vi "Data_Write_Accum.vi"(7 "wfm info":T2, 8 "error in (no error)":errorcluster, 10 "QMH ICR Cluster":T1, 11 "data":i16[](array[numeric])) -> (0 "error out":errorcluster, 1 "Is Accumulated ?":bool, 2 "QMH ICR Cluster":T1, 3 "data":i16[](array[numeric]))   [LabVIEW 2024]
doc: "This VI writes an ACCUMULATED raw dataset to a disk file.\nIf number of accumulations is 1 (i.e. no accumulation), nothing is done, no disk file is created.\nIf number of accumulations > 1 (i.e Nacc > 1) :\n- during the first accumulation, the signal is divided by Nacc and stored into the accumulated disk file.\n- during the next accumulations, the signal is divided by Nacc, added to the previous accumulated signal, and stored into the disk file.\n- the final accumulated signal will contain (signal1 / Nacc + signal2 / Nacc + ... + signalNacc / Nacc)"
uses:
  controls/QMH_ICR_Cluster.ctl
  controls/HARDWARE_Resources.ctl
  controls/PROCESSING_Inputs.ctl
  controls/LOOPS_Inputs.ctl
  controls/OPO_Inputs.ctl
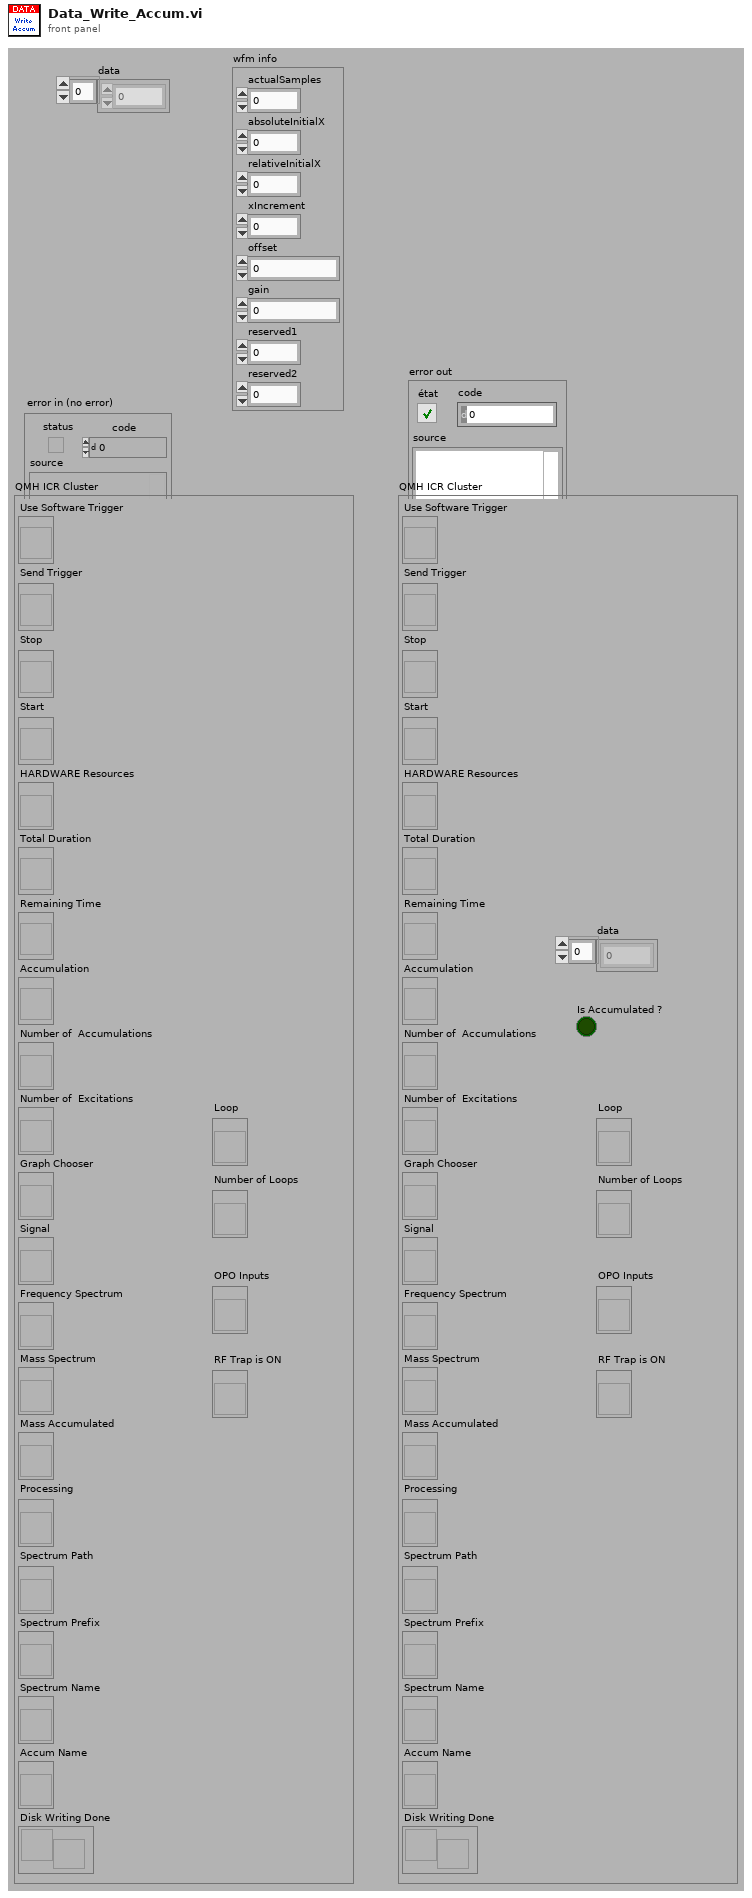
[diagram p1: front panel]
types:
  T1 = typedef "QMH_ICR_Cluster.ctl" = cluster{"Use Software Trigger":refnum<vi>, "Send Trigger":refnum<vi>, "Stop":refnum<vi>, "Start":refnum<vi>, "HARDWARE Resources":refnum<vi>, "Total Duration":refnum<vi>, "Remaining Time":refnum<vi>, "Accumulation":refnum<vi>, "Number of  Accumulations":refnum<vi>, "Number of  Excitations":refnum<vi>, "Graph Chooser":refnum<vi>, "Signal":refnum<vi>, "Frequency Spectrum":refnum<vi>, "Mass Spectrum":refnum<vi>, "Mass Accumulated":refnum<vi>, "Processing":refnum<vi>, "Spectrum Path":refnum<vi>, "Spectrum Prefix":refnum<vi>, "Spectrum Name":refnum<vi>, "Accum Name":refnum<vi>, "Disk Writing Done":refnum<notifier>, "Loop":refnum<vi>, "Number of Loops":refnum<vi>, "OPO Inputs":refnum<vi>, "RF Trap is ON":refnum<vi>}
  T2 = cluster{"actualSamples":i32, "absoluteInitialX":dbl, "relativeInitialX":dbl, "xIncrement":dbl, "offset":dbl, "gain":dbl, "reserved1":dbl, "reserved2":dbl}
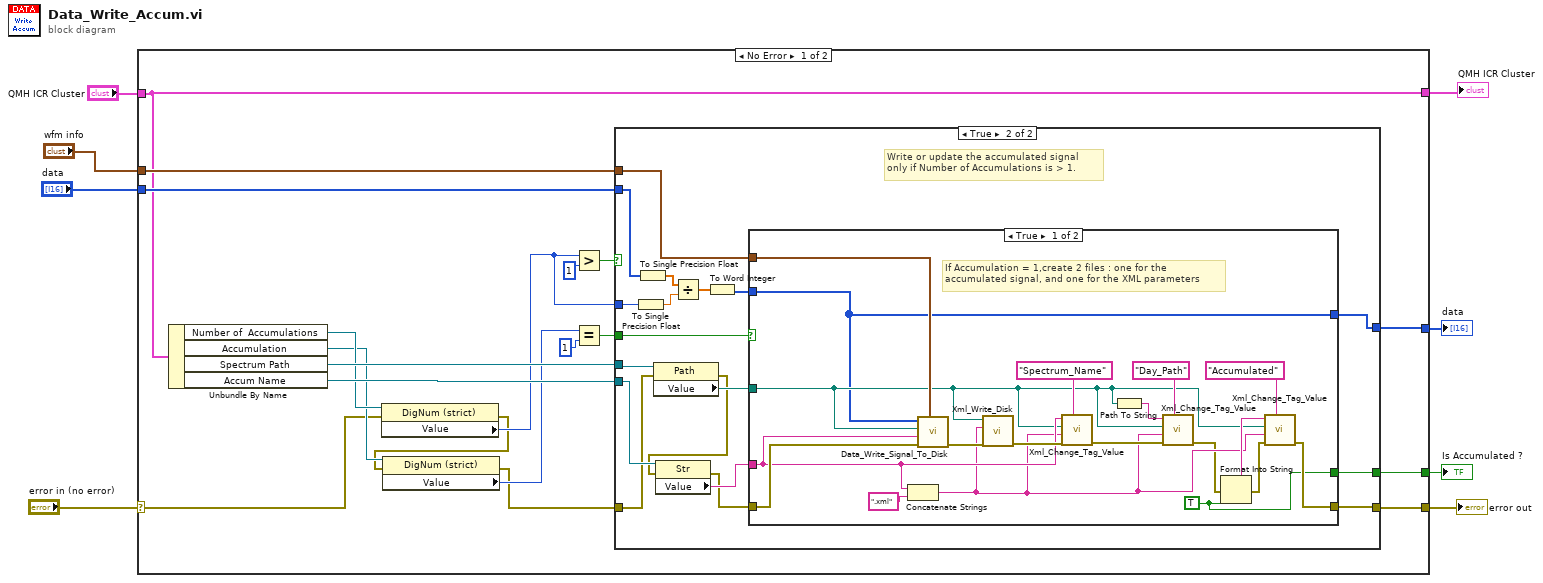
[diagram p0: block diagram]
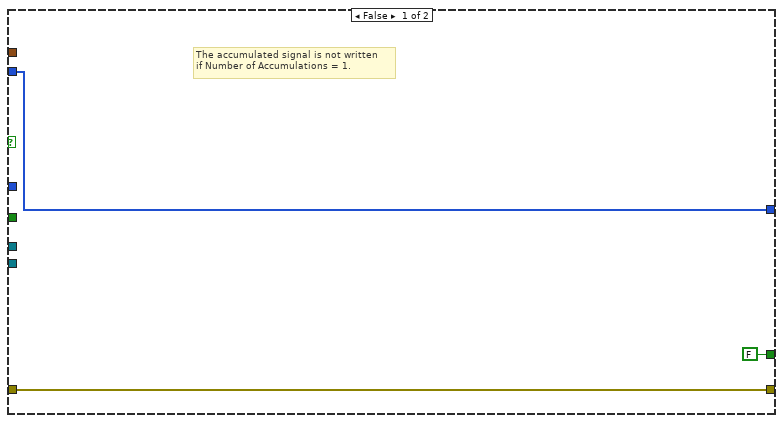
[diagram p2: hidden frame]
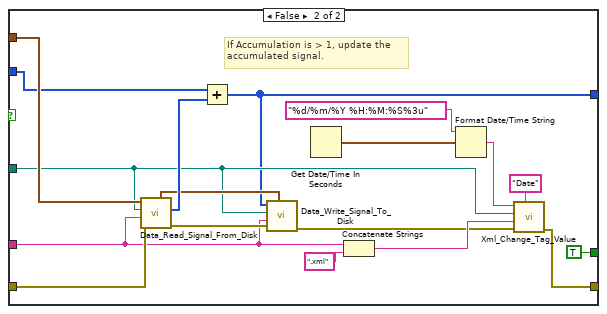
[diagram p3: hidden frame]
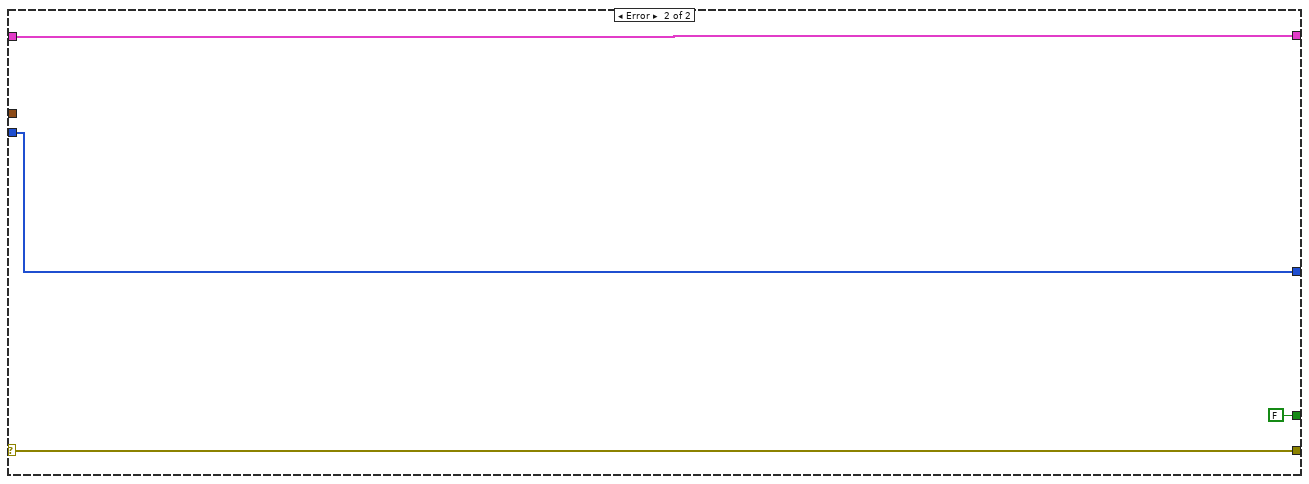
[diagram p4: hidden frame]
diagram:
  n1 = case shown="No Error" "error in (no error)" {
    selector: "error in (no error)" -> [w12 w89]
    tunnel: [w21 w89] -> w6
    tunnel: "wfm info" -> [w27 _]
    tunnel: "data" -> [w26 w87]
    tunnel: "QMH ICR Cluster" -> [w20 w88]
    tunnel: [w20 w88] -> w3
    tunnel: [w13 w87] -> w2
    tunnel: [w9 FALSE] -> w1
    frame No Error {
      n2 = Unbundle By Name(w20) -> ("Number of  Accumulations"=w19:refnum<vi>, "Accumulation"=w18:refnum<vi>, "Spectrum Path"=w25:refnum<vi>, "Accum Name"=w24:refnum<vi>)
      n3 = property class="DigNum (strict)"(reference=w19, error in=w12) -> (error out=w11:errorcluster, "Value"=w14:i16)  [unwired: 1 out]
      n4 = property class="DigNum (strict)"(reference=w18, error in=w11) -> (error out=w10:errorcluster, "Value"=w15:i16)  [unwired: 1 out]
      n5 = Greater?(x=w14, y=i16 1) -> (0:w23:bool)
      n6 = Equal?(x=w15, y=i16 1) -> (x = y?=w16:bool)
      n7 = case shown="True" w23 {
        tunnel: w27 -> [_ w42]
        tunnel: w26 -> [w29 w37]
        tunnel: w25 -> [_ w48]
        tunnel: w24 -> [_ w47]
        tunnel: w10 -> [w30 w40]
        tunnel: [w30 w44] -> w21
        tunnel: w16 -> [_ w43]
        tunnel: w14 -> [_ w41]
        tunnel: [w29 w31] -> w13
        tunnel: [FALSE w32] -> w9
        frame False {
          # "The accumulated signal is not written\nif Number of Accumulations = 1."
        }
        frame True {
          # "Write or update the accumulated signal\nonly if Number of Accumulations is > 1."
          n8 = To Single Precision Float(number=w41) -> (single precision float=w34:sgl)
          n9 = To Single Precision Float(number=w37) -> (single precision float=w35:sgl[])
          n10 = property class="Path"(reference=w48, error in=w40) -> (error out=w39:errorcluster, "Value"=w46:path)  [unwired: 1 out]
          n11 = property class="Str"(reference=w47, error in=w39) -> (error out=w38:errorcluster, "Value"=w45:string)  [unwired: 1 out]
          n12 = Divide(x=w35, y=w34) -> (x/y=w36:sgl[])
          n13 = To Word Integer(number=w36) -> (16bit integer=w33:i16[])
          n14 = case shown="True" w43 {
            tunnel: w46 -> [w54 w78]
            tunnel: w45 -> [w61 w79]
            tunnel: w42 -> [w67 w84]
            tunnel: w38 -> [w66 w85]
            tunnel: [w57 w75] -> w44
            tunnel: w33 -> [w49 w70]
            tunnel: [w50 TRUE] -> w32
            tunnel: [w49 w68] -> w31
            frame True {
              w50 = TRUE
              # "If Accumulation = 1,create 2 files : one for the\naccumulated signal, and one for the XML parameters"
              n15 = Concatenate Strings(w61, ".xml" ("chaîne")) -> (w56:string)
              n16 = call "Data_Write_Signal_To_Disk.vi"("wfm info"=w67, "error in (no error)"=w66, "filename"=w61, "path"=w54, "data"=w49) -> ("error out"=w65:errorcluster)  [unwired: 6 in]
              n17 = call "Xml_Write_Disk.vi"("error in (no error)"=w65, "XML Name"=w56, "Spectrum Path"=w54) -> ("error out"=w62:errorcluster)  [unwired: 7 in, 1 out]
              n18 = call "Xml_Change_Tag_Value.vi"("Tag Name"="Spectrum_Name" ("New Value"), "error in (no error)"=w62, "XML Filename"=w56, "XML Path"=w54, "New Value"=w61) -> ("error out"=w59:errorcluster)  [unwired: 4 in, 2 out]
              n19 = Path To String(path=w54) -> (string=w53:string)
              n20 = call "Xml_Change_Tag_Value.vi"("Tag Name"="Day_Path", "error in (no error)"=w59, "XML Filename"=w56, "XML Path"=w54, "New Value"=w53) -> ("error out"=w52:errorcluster)  [unwired: 4 in, 2 out]
              n21 = Format Into String(error in=w52, w50) -> (resulting string=w58:string, error out=w51:errorcluster)  [unwired: 2 in]
              n22 = call "Xml_Change_Tag_Value.vi"("Tag Name"="Accumulated" ("New Value"), "error in (no error)"=w51, "XML Filename"=w56, "XML Path"=w54, "New Value"=w58) -> ("error out"=w57:errorcluster)  [unwired: 4 in, 2 out]
            }
            frame False {
              # "If Accumulation is > 1, update the\naccumulated signal."
              n23 = call "Data_Read_Signal_From_Disk.vi"("error in (no error)"=w85, "filename"=w79, "path"=w78, "wfm info"=w84) -> ("error out"=w82:errorcluster, "data"=w83:i16[], "wfm info"=w81:T2)  [unwired: 4 in, 1 out]
              n24 = Add(x=w70, y=w83) -> (x+y=w68:i16[])
              n25 = call "Data_Write_Signal_To_Disk.vi"("wfm info"=w81, "error in (no error)"=w82, "filename"=w79, "path"=w78, "data"=w68) -> ("error out"=w76:errorcluster)  [unwired: 6 in]
              n26 = Get Date/Time In Seconds() -> (seconds since 1Jan1904=w73:timestamp)
              n27 = Concatenate Strings(w79, ".xml" ("chaîne")) -> (w77:string)
              n28 = Format Date/Time String(time format string (%c)="%d/%m/%Y %H:%M:%S%3u" ("chaîne de format de l'heure (%c)"), seconds (now)=w73) -> (date/time string=w72:string)  [unwired: 1 in]
              n29 = call "Xml_Change_Tag_Value.vi"("Tag Name"="Date", "error in (no error)"=w76, "XML Filename"=w77, "XML Path"=w78, "New Value"=w72) -> ("error out"=w75:errorcluster)  [unwired: 4 in, 2 out]
            }
          }
        }
      }
    }
    frame Error {
    }
  }
  "error out" <- w6
  "QMH ICR Cluster" <- w3
  "data" <- w2
  "Is Accumulated ?" <- w1
